vi "ngi set adjustable parameters.vi"(7 "node nummer":i32=1, 8 "error in":errorcluster, 10 "dust mac adress":string[](array[string])=["\u0000\u0017\r\u0000\u0000`\u001a½", "\u0000\u0017\r\u0000\u0000`)š", "\u0000\u0017\r\u0000\u0000`$«", "\u0000\u0017\r\u0000\u0000` ÿ"], 11 "Adjustable Parameters":T1(array[cluster])) -> (0 "error out":errorcluster)   [LabVIEW 2017]
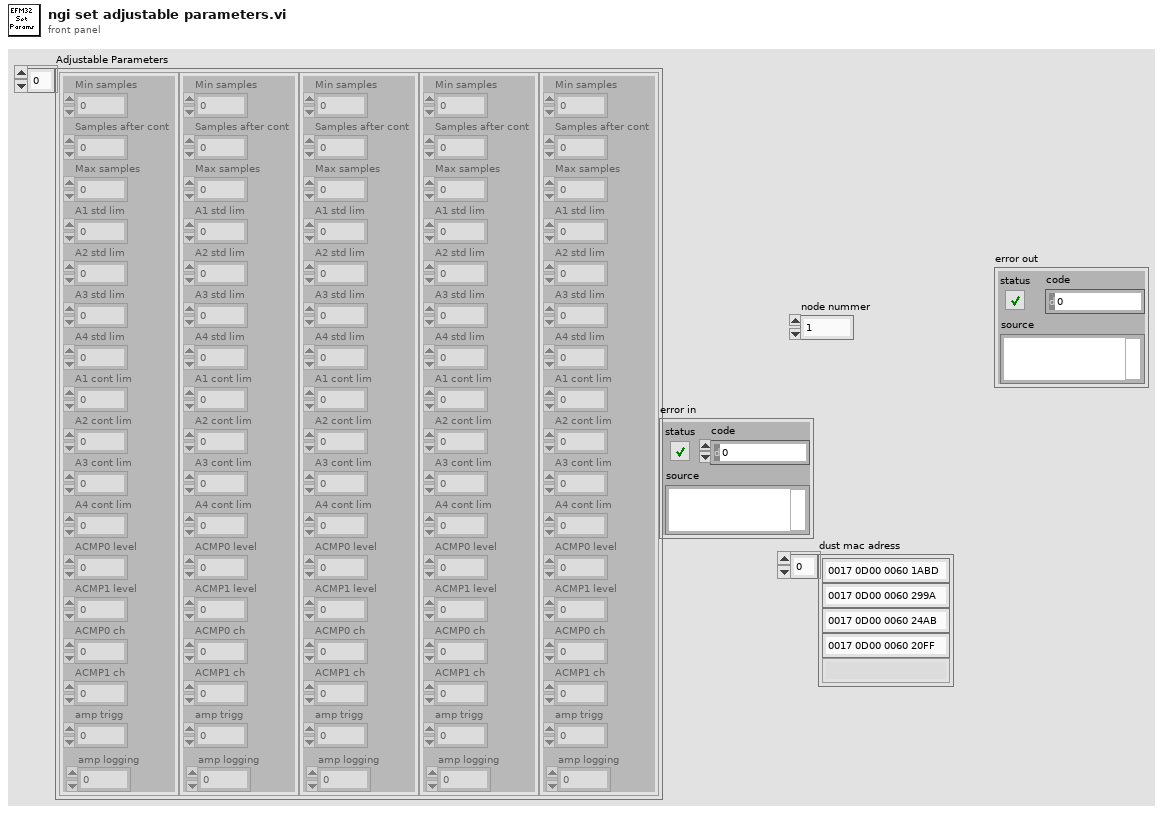
[diagram p1: front panel]
types:
  T1 = cluster{"Min samples":u32, "Samples after cont":u32, "Max samples":u32, "A1 std lim":sgl, "A2 std lim":sgl, "A3 std lim":sgl, "A4 std lim":sgl, "A1 cont lim":sgl, "A2 cont lim":sgl, "A3 cont lim":sgl, "A4 cont lim":sgl, "ACMP0 level":u32, "ACMP1 level":u32, "ACMP0 ch":u8, "ACMP1 ch":u8, "amp trigg":u16, "amp logging":u16}[]
  T2 = enum16{"big-endian, network order", "native, host order", "little-endian"}
  T3 = cluster{"Min samples":u32, "Samples after cont":u32, "Max samples":u32, "A1 std lim":sgl, "A2 std lim":sgl, "A3 std lim":sgl, "A4 std lim":sgl, "A1 cont lim":sgl, "A2 cont lim":sgl, "A3 cont lim":sgl, "A4 cont lim":sgl, "ACMP0 level":u32, "ACMP1 level":u32, "ACMP0 ch":u8, "ACMP1 ch":u8, "amp trigg":u16, "amp logging":u16}
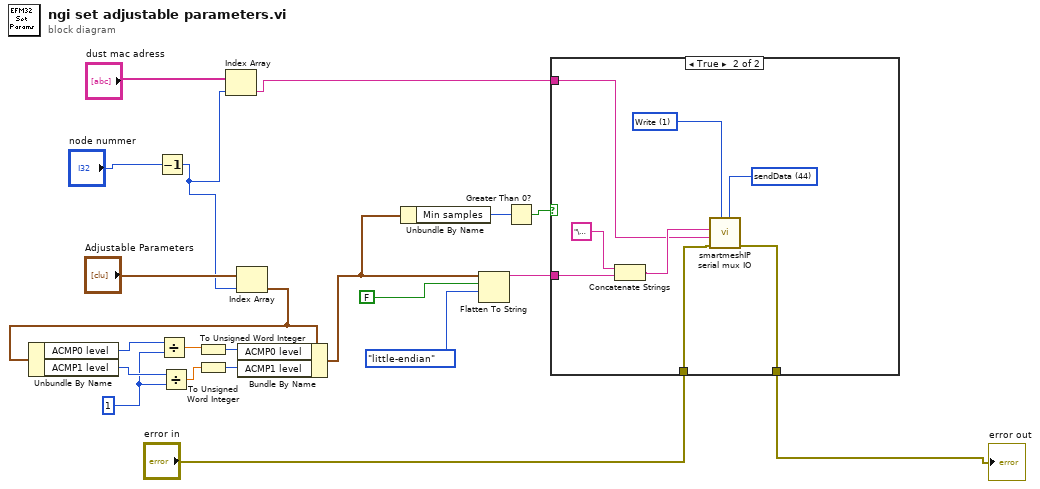
[diagram p0: block diagram]
diagram:
  w1 = u32 1 ("y")
  n1 = Decrement(x="node nummer") -> (x-1=w10:i32)
  n2 = Index Array(array="dust mac adress", index=w10) -> (element=w13:string)
  n3 = Index Array(array="Adjustable Parameters", index=w10) -> (element=w9:T3)
  n4 = Unbundle By Name(w9) -> ("ACMP0 level"=w3:u32, "ACMP1 level"=w2:u32)
  n5 = Divide(x=w3, y=w1) -> (x/y=w5:dbl)
  n6 = Divide(x=w2, y=w1) -> (x/y=w4:dbl)
  n7 = To Unsigned Word Integer(number=w5) -> (unsigned 16bit integer=w7:u16)
  n8 = To Unsigned Word Integer(number=w4) -> (unsigned 16bit integer=w6:u16)
  n9 = Bundle By Name(cluster=w9, "ACMP0 level"=w7, "ACMP1 level"=w6) -> (w8:T3)
  n10 = Unbundle By Name(w8) -> ("Min samples"=w19:u32)
  n11 = Flatten To String(anything=w8, prepend array or string size? (T)=FALSE, byte order (0:big-endian, network order)=T2."little-endian") -> (data string=w20:string)  [unwired: 1 in, 2 out]
  n12 = Greater Than 0?(x=w19) -> (x > 0?=w21:bool)
  n13 = case shown="True" w21 {
    tunnel: w20 -> [_ w28]
    tunnel: "error in" -> [w22 w25]
    tunnel: [w22 w24] -> w16
    tunnel: w13 -> [_ w23]
    frame False {
    }
    frame True {
      w29 = u8 44 items=["subscribe"=22, "startNetwork"=45, "setUser"=58, "setTime"=54, "setNetworkConfig"=26, "setLicense"=56, "setIPConfig"=68, "setDownstreamFrameMode"=51, "setCommonJoinKey"=66, "setAdvertising"=50, "setACLEntry"=39, "sendIP"=59, "sendData"=44, "restorFactoryDefaults"=61, "reset"=21, "radiotestTx"=35, "radiotestRx"=37, "pingMote"=42, "getTime"=23, "getSystemInfo"=46, "radiotestStatistics"=38, "getPathInfo"=48, "getNextPath"=49, "getNextACLEntry"=40, "getNetworkInfo"=64, "getNetworkConfig"=63, "getMoteLinks"=70, "getMoteInfo"=62, "getMoteConfigByld"=65, "getMoteConfig"=47, "getManagerStatistics"=53, "getLog"=43, "getLicense"=55, "getIPConfig"=67, "exchangeNetworkID"=34, "exchangeMoteJoinKey"=33, "deleteMote"=69, "deleteACLEntry"=41, "clearStatistics"=31] ("commandType_write")
      w30 = u16 1 items=["Connect", "Write", "Read", "Close"] ("State")
      n14 = Concatenate Strings("\u0006" ("string"), w28) -> (w27:string)
      n15 = call "smartmeshIP serial mux IO.vi"("tx_commandType"=w29, "State"=w30, "error in"=w25, "MAC source"=w23, "tx_data"=w27) -> ("error out"=w24:errorcluster)  [unwired: 1 in, 5 out]
    }
  }
  "error out" <- w16
